vi "Команда обмена 86 (принудительный шаг вперед ) (SubVI).vi"(7 "error in":errorcluster, 9 "TCP connection ID":refnum<k5>) -> (27 "error out":errorcluster)   [LabVIEW 2013]
doc: "Команда 85 - инициировать запрос на обновление параметров мишени с переданным id"
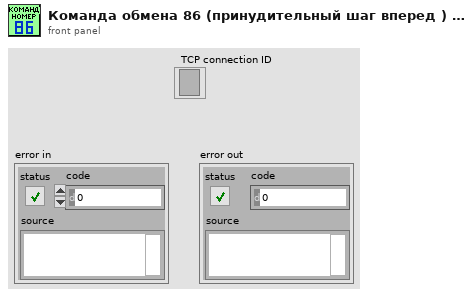
[diagram p1: front panel]
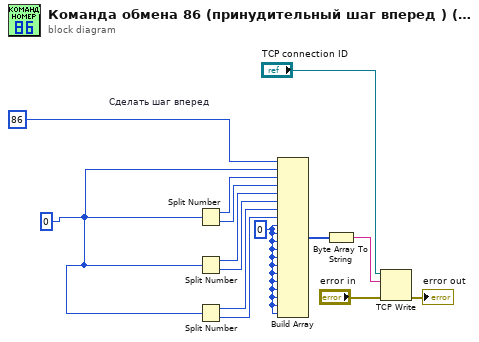
[diagram p0: block diagram]
diagram:
  w1 = u16 0 ("element")
  w14 = u16 0 ("element")
  w3 = u8 86  # Сделать шаг вперед
  n1 = Split Number(x=w1) -> (hi(x)=w8:u8, lo(x)=w9:u8)
  n2 = Split Number(x=w1) -> (hi(x)=w12:u8, lo(x)=w13:u8)
  n3 = Split Number(x=w1) -> (hi(x)=w10:u8, lo(x)=w11:u8)
  n4 = Build Array(w3, w1, w8, w9, w12, w13, w10, w11, w14, w14, w14, w14, w14, w14, w14, w14, w14, w14, w14, w14) -> (w4:u16[])
  n5 = Byte Array To String(unsigned byte array=w4) -> (string=w6:string)
  n6 = TCP Write(connection ID="TCP connection ID", data in=w6, error in (no error)="error in") -> (error out=→"error out":errorcluster)  [unwired: 1 in, 2 out]
